vi "Create Data Server.vi"(5 "data server options":T1={"Enable Data Server"=FALSE, "Period"=100} {"Period" format="%d ms"}, 7 "Framework Configuration":refnum<class "Framework Configuration.lvclass">, 8 "error in (no error)":errorcluster, 10 "Plugins":refnum<class "Plugin.lvclass">[](array[class]), 11 "Framework in":refnum<class "Framework.lvclass">) -> (0 "error out":errorcluster, 2 "Data Server Thread":refnum<class "Data Server Thread.lvclass">, 3 "Framework out":refnum<class "Framework.lvclass">)   [LabVIEW 2021, in "DSF Core.lvlib" / "Framework.lvclass"]
uses:
  Framework.lvclass
  Plugin/Plugin.lvclass
  Thread/Data Server/Data Server Thread.lvclass
  C:/dev/git/custom-devices/niveristand-data-sharing-framework-custom-device/Source/Core/Classes/Thread/Thread.lvclass
  Data Server Options.ctl
  Configuration/Core/Framework/Framework Configuration.lvclass
  Thread/Data Server/Framework.ctl
  Status/Status Pointer.lvclass
  Thread/Data Server/Plugin.ctl
  Thread/Data Server/Group.ctl
  Buffers/Buffers.lvclass
  Transfer/Transfer.lvclass
  Framework Status/Framework Status.lvclass/Framework Status.ctl
  Plugin/Plugin.lvclass/Plugin.ctl
  Transfer Group/Transfer Group.lvclass/Transfer Group.ctl
  Thread/Thread.lvclass/Thread.ctl
  Interface/Interface.lvclass/Interface.ctl
  Thread/Data Server/Data Server Thread.lvclass/Data Server Thread.ctl
  Framework.lvclass/Framework.ctl
  Interface/Plugin/Create.vi
  Thread/Set Name.vi
  Thread/Set Thread Parameters.vi
  Transfer Group/Get ID.vi
  Interface/New Interface.vi
  Interface/Create RT FIFO.vi
  Interface/Plugin/Plugin Interface.lvclass
  C:/dev/git/custom-devices/niveristand-data-sharing-framework-custom-device/Source/Core/Classes/Interface/Interface.lvclass
  Transfer Group/Transfer Group.lvclass
  Framework Status/Framework Status.lvclass
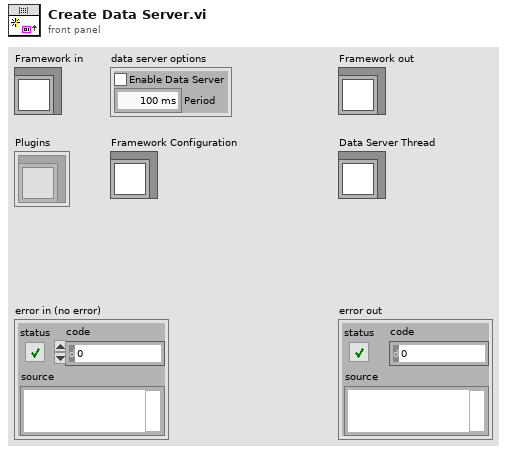
[diagram p1: front panel]
types:
  T1 = typedef "DSF Core.lvlib/Framework.lvclass/Data Server Options.ctl" = cluster{"Enable Data Server":bool, "Period":u32}
  T2 = typedef "DSF Core.lvlib/Data Server Thread.lvclass/Framework.ctl" = cluster{"Framework Status":refnum<class "Status Pointer.lvclass">, "Plugins":T3[]}
  T3 = typedef "DSF Core.lvlib/Data Server Thread.lvclass/Plugin.ctl" = cluster{"Plugin Status":refnum<class "Status Pointer.lvclass">, "Groups":T4[]}
  T4 = typedef "DSF Core.lvlib/Data Server Thread.lvclass/Group.ctl" = cluster{"Group Buffers":refnum<class "Buffers.lvclass">, "Group Status":refnum<class "Status Pointer.lvclass">, "Transfers":refnum<class "Transfer.lvclass">[]}
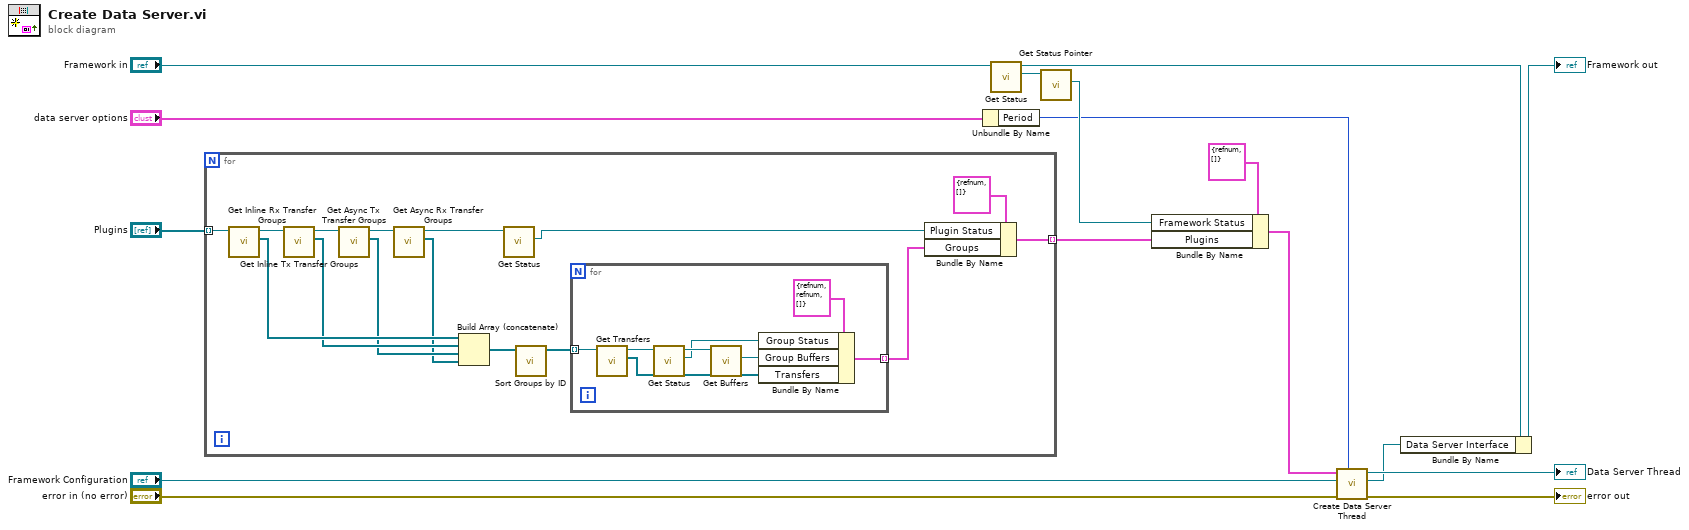
[diagram p0: block diagram]
diagram:
  n1 = for {
    tunnel: "Plugins" -> [w29] mode=indexing
    tunnel: [w30] -> w7 mode=indexing
    n2 = call "Get Inline Rx Transfer Groups.vi"("Plugin in"=w29) -> ("Inline Rx Transfer Groups"=w25:refnum<class "Transfer Group.lvclass">[], "Plugin out"=w28:refnum<class "Plugin.lvclass">)  [unwired: 9 in]
    n3 = call "Get Inline Tx Transfer Groups.vi"("Plugin in"=w28) -> ("Inline Tx Transfer Groups"=w24:refnum<class "Transfer Group.lvclass">[], "Plugin out"=w27:refnum<class "Plugin.lvclass">)  [unwired: 9 in]
    n4 = call "Get Async Tx Transfer Groups.vi"("Plugin in"=w27) -> ("Async Tx Transfer Groups"=w23:refnum<class "Transfer Group.lvclass">[], "Plugin out"=w26:refnum<class "Plugin.lvclass">)  [unwired: 9 in]
    n5 = call "Get Async Rx Transfer Groups.vi"("Plugin in"=w26) -> ("Async Rx Transfer Groups"=w21:refnum<class "Transfer Group.lvclass">[], "Plugin out"=w18:refnum<class "Plugin.lvclass">)  [unwired: 9 in]
    n6 = Build Array (concatenate)(w25, w24, w23, w21) -> (w22:refnum<class "Transfer Group.lvclass">[])
    n7 = call "Get Status.vi"("Plugin in"=w18) -> ("status pointer"=w17:refnum<class "Status Pointer.lvclass">)  [unwired: 9 in, 1 out]
    n8 = call "Sort Groups by ID.vi"("Transfers Groups in"=w22) -> ("ID-sorted Transfers Groups out"=w20:refnum<class "Transfer Group.lvclass">[])  [unwired: 9 in, 1 out]
    n9 = for {
      tunnel: w20 -> [w36] mode=indexing
      tunnel: [w37] -> w19 mode=indexing
      n10 = call "Get Transfers.vi"("Transfer Group in"=w36) -> ("Transfers"=w35:refnum<class "Transfer.lvclass">[], "Transfer Group out"=w34:refnum<class "Transfer Group.lvclass">)  [unwired: 9 in]
      n11 = call "Get Status.vi"("Transfer Group in"=w34) -> ("status pointer"=w32:refnum<class "Status Pointer.lvclass">, "Transfer Group out"=w33:refnum<class "Transfer Group.lvclass">)  [unwired: 9 in]
      n12 = call "Get Buffers.vi"("Transfer Group in"=w33) -> ("Buffers"=w38:refnum<class "Buffers.lvclass">)  [unwired: 9 in, 1 out]
      n13 = Bundle By Name(cluster=T4 {"Group Buffers"=refnum, "Group Status"=refnum, "Transfers"=[]} ("Group"), "Group Status"=w32, "Group Buffers"=w38, "Transfers"=w35) -> (w37:T4)
    }
    n14 = Bundle By Name(cluster=T3 {"Plugin Status"=refnum, "Groups"=[]} ("Plugin"), "Plugin Status"=w17, "Groups"=w19) -> (w30:T3)
  }
  n15 = Unbundle By Name("data server options") -> ("Period"=w1:u32)
  n16 = call "Get Status.vi"("Framework in"="Framework in") -> ("Status"=w4:refnum<class "Framework Status.lvclass">, "Framework out"=w2:refnum<class "Framework.lvclass">)  [unwired: 9 in]
  n17 = call "Get Status Pointer.vi"("Framework Status in"=w4) -> ("status pointer"=w3:refnum<class "Status Pointer.lvclass">)  [unwired: 8 in, 2 out]
  n18 = Bundle By Name(cluster=T2 {"Framework Status"=refnum, "Plugins"=[]} ("Buffers"), "Framework Status"=w3, "Plugins"=w7) -> (w6:T2)
  n19 = call "Create Data Server Thread.vi"("period (100 ms)"=w1, "error in (no error)"="error in (no error)", "Framework Configuration"="Framework Configuration", "Buffers"=w6) -> ("error out"=→"error out":errorcluster, "Interface"=w11:refnum<class "Plugin Interface.lvclass">, "Data Server Thread out"=→"Data Server Thread":refnum<class "Data Server Thread.lvclass">)  [unwired: 5 in]
  n20 = Bundle By Name(cluster=w2, "Data Server Interface"=w11) -> (→"Framework out":refnum<class "Framework.lvclass">)
